vi "RegisterUserEvents.vi"(8 "error in (no error)":errorcluster) -> (0 "error out":errorcluster, 3 "Event Registration Refnum":refnum<event-registration>)   [LabVIEW 2015, in "ESLSCDLL.lvlib"]
uses:
  ESLSCDLL.lvlib
  Globals.vi
panel:
  out "Path":path
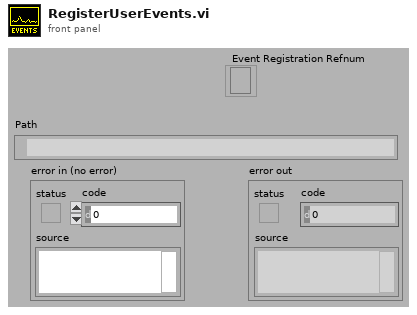
[diagram p1: front panel]
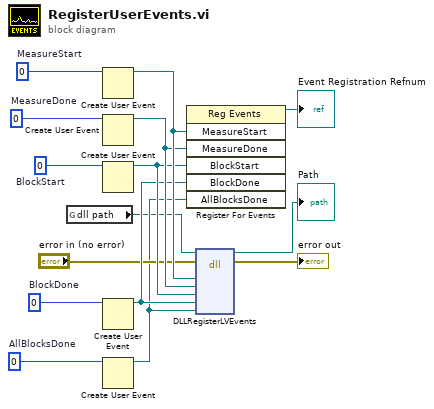
[diagram p0: block diagram]
diagram:
  w4 = 0  # AllBlocksDone
  w12 = 0  # BlockStart
  w7 = 0  # MeasureStart
  w13 = 0  # BlockDone
  w15 = 0  # MeasureDone
  n1 = global read "Globals.vi" "dll path"() -> (w1:path)
  n2 = Create User Event(user event datatype=w7) -> (user event=w11:refnum<user-event>)  [unwired: 1 in, 1 out]
  n3 = Create User Event(user event datatype=w15) -> (user event=w10:refnum<user-event>)  [unwired: 1 in, 1 out]
  n4 = Create User Event(user event datatype=w12) -> (user event=w9:refnum<user-event>)  [unwired: 1 in, 1 out]
  n5 = Create User Event(user event datatype=w13) -> (user event=w8:refnum<user-event>)  [unwired: 1 in, 1 out]
  n6 = Create User Event(user event datatype=w4) -> (user event=w3:refnum<user-event>)  [unwired: 1 in, 1 out]
  n7 = register-events(w11, w10, w9, w8, w3) -> (reference out=→"Event Registration Refnum":refnum<event-registration>)  [unwired: 2 in, 1 out]
  n8 = dll-call lib="C:/Users/Gerhard/ENTW/PCIE/64bit/lv64/board.vis/ESLSCDLL.dll" fn="DLLRegisterLVEvents" ("lwlscdll.dll:DLLWriteLongS0")(path in=w1, error in="error in (no error)", "measureStartEvent"=w11, "measureDoneEvent"=w10, "blockStartEvent"=w9, "blockDoneEvent"=w8, "allBlocksDoneEvent"=w3) -> (path out=→"Path":path, error out=→"error out":errorcluster)  [unwired: 7 in]
